vi "niDTS BT Rx Test UTIL BT TX Parameters to BDR Parameters.vi"(7 "Default Parameters":T8={"Channel"=3, "Dut Tx Power"=0.0, "External Attenuation (dB)"=[0.0], "Data Rate"=enum."1", "Packet type"=enum."DH1", "Payload Data"=enum."PN9", "Carrier Mode"=enum."Burst", "Number of Packets"=1500, "Report Period (ms)"=1000.0, "BD ADDRESS"=0, "Dirty Tx"=FALSE, "Corrupt Alternate CRC"=FALSE, "Packet Header"={"LT Address"=0, "Flow"=0, "ARQN"=enum."NAK", "Sequence Bit"=0}, "Payload Header"={"LCh"=0, "HeaderFlowControlBit"=FALSE, "Length (-1 AutoSet Max)"=-1}, "Trigger"={"TriggerEdge"=enum."RISing", "TriggerSource"=enum."IMMediate", "TriggerDelay (sec)"=0.0, "TriggerTimeout (sec)"=0.0}} {"BD ADDRESS" max=16777215 format="%.0x"}) -> (8 "BT BDR Parameters":T1={"Channel"=3, "Tx Power (dBm) "=0.0, "External Attenuation (dB)"=0.0, "BDR Packet type"=enum."DH1", "Payload Data"=enum."PN9", "Carrier Mode"=enum."Burst", "Number of Packets"=1500, "Report Period (ms)"=1000.0, "BD ADDRESS"="", "Packet Header"={"LT Address"=0, "Flow"=0, "ARQN"=enum."NAK", "Sequence Bit"=0}, "Dirty Packets"=FALSE, "Corrupt Alternate CRC"=FALSE, "Payload Header"={"LCh"=0, "HeaderFlowControlBit"=FALSE, "Length (-1 AutoSet Max)"=-1}, "Trigger"={"TriggerEdge"=enum."RISing", "TriggerSource"=enum."IMMediate", "TriggerDelay (sec)"=0.0, "TriggerTimeout (sec)"=0.0}})   [LabVIEW 2014, in "niDTS BT.lvlib"]
uses:
  niDTS BT.lvlib
  Rx Test/Includes/niDTS BT Rx Test INC Parameters.ctl
  Includes/niDTS BT INC Packet Type.ctl
  Tx Test/Includes/niDTS BT Tx Test INC BD Payload Data.ctl
  Rx Test/Includes/niDTS BT Rx Test INC Carrier Mode.ctl
  Rx Test/Includes/niDTS BT Rx Test INC Packet Header.ctl
  Rx Test/Includes/niDTS BT Rx Test INC Payload Header.ctl
  Includes/niDTS BT DUT INC SG Trigger.ctl
  Includes/niDTS BT BDR Rx Test INC Parameters.ctl
  BDR Tx Test/Includes/niDTS BT INC BDR Packet Type.ctl
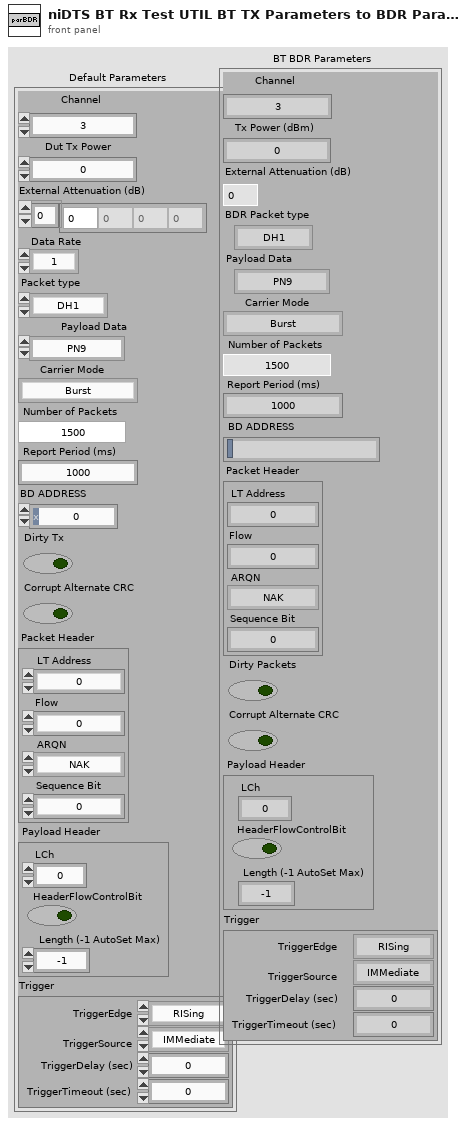
[diagram p1: front panel]
types:
  T1 = typedef "niDTS BT.lvlib/niDTS BT BDR Rx Test INC Parameters.ctl" = cluster{"Channel":i32, "Tx Power (dBm) ":dbl, "External Attenuation (dB)":dbl, "BDR Packet type":T2, "Payload Data":T3, "Carrier Mode":T4, "Number of Packets":i32, "Report Period (ms)":dbl, "BD ADDRESS":string, "Packet Header":T5, "Dirty Packets":bool, "Corrupt Alternate CRC":bool, "Payload Header":T6, "Trigger":T7}
  T2 = typedef "niDTS BT.lvlib/niDTS BT INC BDR Packet Type.ctl" = enum16{"NULL", "POLL", "FHS", "DM1", "DH1", "HV1", "HV2", "HV3", "EV3", "DV", "AUX1", "DM3", "DH3", "EV4", "EV5", "DM5", "DH5"}
  T3 = typedef "niDTS BT.lvlib/niDTS BT Tx Test INC BD Payload Data.ctl" = enum16{"0", "1", "01", "00001111", "PN9", "AUTO"}
  T4 = typedef "niDTS BT.lvlib/niDTS BT Rx Test INC Carrier Mode.ctl" = enum16{"Burst", "Continuous"}
  T5 = typedef "niDTS BT.lvlib/niDTS BT Rx Test INC Packet Header.ctl" = cluster{"LT Address":i8, "Flow":i8, "ARQN":enum16{"NAK", "ACK"}, "Sequence Bit":i8}
  T6 = typedef "niDTS BT.lvlib/niDTS BT Rx Test INC Payload Header.ctl" = cluster{"LCh":i32, "HeaderFlowControlBit":bool, "Length (-1 AutoSet Max)":i32}
  T7 = typedef "niDTS BT.lvlib/niDTS BT DUT INC SG Trigger.ctl" = cluster{"TriggerEdge":enum16{"RISing", "FALLing"}, "TriggerSource":enum16{"IMMediate", "PFI 0", "PFI 1", "RTSI 0", "RTSI 1", "RTSI 2", "RTSI 3", "RTSI 4", "RTSI 5", "RTSI 6", "RTSI 7", "PXI STAR", "Software"}, "TriggerDelay (sec)":dbl, "TriggerTimeout (sec)":dbl}
  T8 = typedef "niDTS BT.lvlib/niDTS BT Rx Test INC Parameters.ctl" = cluster{"Channel":i32, "Dut Tx Power":dbl, "External Attenuation (dB)":dbl[], "Data Rate":enum16{"1", "2", "3"}, "Packet type":T9, "Payload Data":T3, "Carrier Mode":T4, "Number of Packets":i32, "Report Period (ms)":dbl, "BD ADDRESS":i64, "Dirty Tx":bool, "Corrupt Alternate CRC":bool, "Packet Header":T5, "Payload Header":T6, "Trigger":T7}
  T9 = typedef "niDTS BT.lvlib/niDTS BT INC Packet Type.ctl" = enum16{"NULL", "POLL", "FHS", "DM1", "DH1", "HV1", "HV2", "HV3", "EV3", "DV", "AUX1", "DM3", "DH3", "EV4", "EV5", "DM5", "DH5", "LE-TP"}
  T10 = enum16{"NULL", "POLL", "FHS", "DM1", "DH1", "HV1", "HV2", "HV3", "EV3", "DV", "AUX1", "DM3", "DH3", "EV4", "EV5", "DM5", "DH5"}
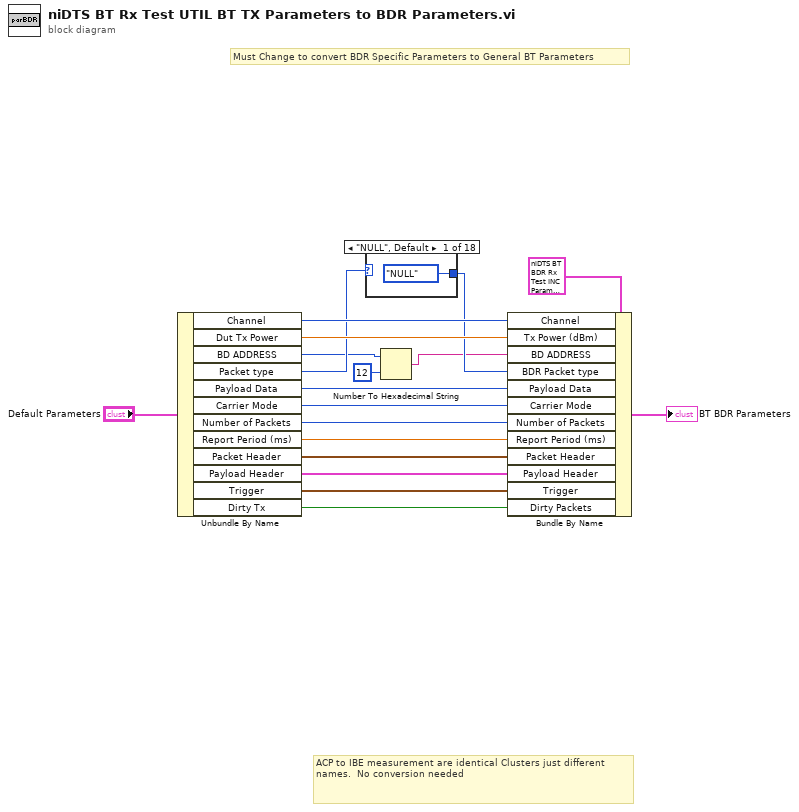
[diagram p0: block diagram]
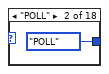
[diagram p2: hidden frame]
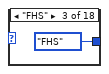
[diagram p3: hidden frame]
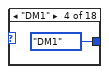
[diagram p4: hidden frame]
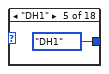
[diagram p5: hidden frame]
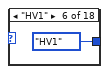
[diagram p6: hidden frame]
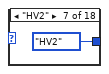
[diagram p7: hidden frame]
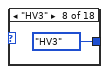
[diagram p8: hidden frame]
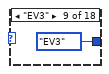
[diagram p9: hidden frame]
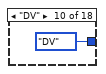
[diagram p10: hidden frame]
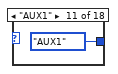
[diagram p11: hidden frame]
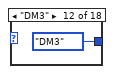
[diagram p12: hidden frame]
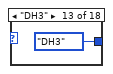
[diagram p13: hidden frame]
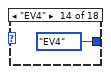
[diagram p14: hidden frame]
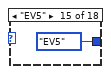
[diagram p15: hidden frame]
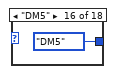
[diagram p16: hidden frame]
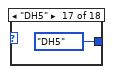
[diagram p17: hidden frame]
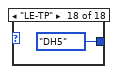
[diagram p18: hidden frame]
diagram:
  # "ACP to IBE measurement are identical Clusters just different names.  No conversion needed"
  # "Must Change to convert BDR Specific Parameters to General BT Parameters"
  n1 = Unbundle By Name("Default Parameters") -> ("Channel"=w16:i32, "Dut Tx Power"=w15:dbl, "BD ADDRESS"=w3:i64, "Packet type"=w14:T9, "Payload Data"=w12:T3, "Carrier Mode"=w11:T4, "Number of Packets"=w10:i32, "Report Period (ms)"=w9:dbl, "Packet Header"=w8:T5, "Payload Header"=w7:T6, "Trigger"=w6:T7, "Dirty Tx"=w1:bool)
  n2 = case shown="\"NULL\", Default" w14 {
    tunnel: [T10."NULL" T10."POLL" T10."FHS" T10."DM1" T10."DH1" T10."HV1" T10."HV2" T10."HV3" T10."EV3" T10."DV" T10."AUX1" T10."DM3" T10."DH3" T10."EV4" T10."EV5" T10."DM5" T10."DH5" T10."DH5"] -> w13
    frame "NULL", Default {
    }
    frame "POLL" {
    }
    frame "FHS" {
    }
    frame "DM1" {
    }
    frame "DH1" {
    }
    frame "HV1" {
    }
    frame "HV2" {
    }
    frame "HV3" {
    }
    frame "EV3" {
    }
    frame "DV" {
    }
    frame "AUX1" {
    }
    frame "DM3" {
    }
    frame "DH3" {
    }
    frame "EV4" {
    }
    frame "EV5" {
    }
    frame "DM5" {
    }
    frame "DH5" {
    }
    frame "LE-TP" {
    }
  }
  n3 = Number To Hexadecimal String(1:i16 12 ("width (-)"), 2:w3) -> (0:w2:string)
  n4 = Bundle By Name(cluster=T1 {"Channel"=1, "Tx Power (dBm) "=-80.0, "External Attenuation (dB)"=0.0, "BDR Packet type"=enum."DH1", "Payload Data"=enum."PN9", "Carrier Mode"=enum."Burst", "Number of Packets"=-1, "Report Period (ms)"=500.0, "BD ADDRESS"="", "Packet Header"={"LT Address"=0, "Flow"=0, "ARQN"=enum."NAK", "Sequence Bit"=0}, "Dirty Packets"=FALSE, "Corrupt Alternate CRC"=FALSE, "Payload Header"={"LCh"=7, "HeaderFlowControlBit"=FALSE, "Length (-1 AutoSet Max)"=-1}, "Trigger"={"TriggerEdge"=enum."RISing", "TriggerSource"=enum."IMMediate", "TriggerDelay (sec)"=0.0, "TriggerTimeout (sec)"=0.0}} ("BT BDR Parameters 2"), "Channel"=w16, "Tx Power (dBm)"=w15, "BD ADDRESS"=w2, "BDR Packet type"=w13, "Payload Data"=w12, "Carrier Mode"=w11, "Number of Packets"=w10, "Report Period (ms)"=w9, "Packet Header"=w8, "Payload Header"=w7, "Trigger"=w6, "Dirty Packets"=w1) -> (→"BT BDR Parameters":T1)
